vi "launch_main.vi"(8 "error in (no error)":errorcluster, 9 "enable_event":bool, 10 "queue_size":i32=10, 11 "run_f_stop_t":bool) -> (0 "error out":errorcluster, 3 "references":T1)   [LabVIEW 2015, in "repub-dvr_nre.lvlib"]
uses:
  repub-dvr_nre.lvlib
  public/_controls/references.ctl
  _controls/input.ctl
  _controls/input_command.ctl
  _controls/output.ctl
  _controls/data.ctl
  public/_controls/configuration.ctl
  public/_controls/change.ctl
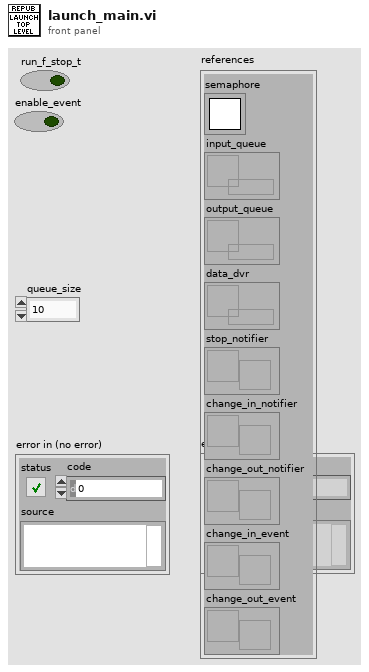
[diagram p1: front panel]
types:
  T1 = typedef "repub-dvr_nre.lvlib/references.ctl" = cluster{"semaphore":T2, "input_queue":refnum<queue>, "output_queue":refnum<queue>, "data_dvr":refnum<data-value>, "stop_notifier":refnum<notifier>, "change_in_notifier":refnum<notifier>, "change_out_notifier":refnum<notifier>, "change_in_event":refnum<user-event>, "change_out_event":refnum<user-event>}
  T2 = typedef "Semaphore RefNum" = refnum<k1>
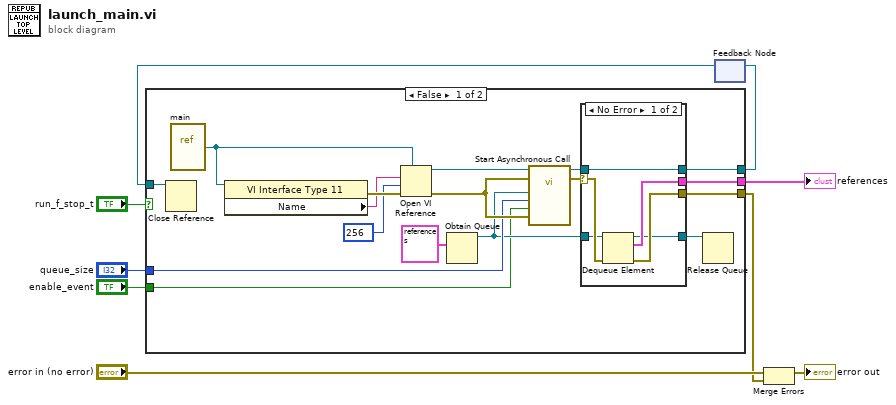
[diagram p0: block diagram]
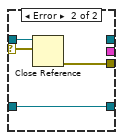
[diagram p2: hidden frame]
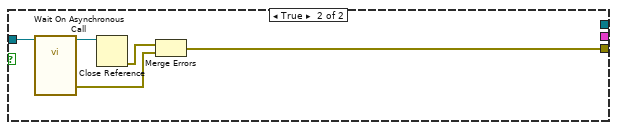
[diagram p3: hidden frame]
diagram:
  n1 = feedback #1() -> (w7:refnum<vi>)  [unwired: 1 in]
  n2 = case shown="False" "run_f_stop_t" {
    tunnel: [w21 _] -> w8
    tunnel: w7 -> [w19 w40]
    tunnel: [w20 w37] -> w5
    tunnel: [w15 _] -> w3
    tunnel: "queue_size" -> [w13 _]
    tunnel: "enable_event" -> [w10 _]
    frame False {
      n3 = Close Reference(reference=w19) -> ()  [unwired: 1 in, 1 out]
      n4 = vi-ref "main.vi"() -> (w18:refnum<vi>)
      n5 = property class="VI Interface Type 11"(reference=w18) -> (error out=w26:errorcluster, "Name"=w25:string)  [unwired: 1 in, 1 out]
      n6 = Open VI Reference(type specifier VI Refnum (for type only)=w18, vi path=w25, options=256, error in (no error)=w26) -> (vi reference=w17:refnum<vi>, error out=w14:errorcluster)  [unwired: 2 in]
      n7 = Obtain Queue(element data type=T1 {"semaphore"=refnum, "input_queue"=refnum, "output_queue"=refnum, "data_dvr"=refnum, "stop_notifier"=refnum, "change_in_notifier"=refnum, "change_out_notifier"=refnum, "change_in_event"=refnum, "change_out_event"=refnum} ("references")) -> (queue out=w12:refnum<queue>)  [unwired: 4 in, 2 out]
      n8 = call-by-ref "Start Asynchronous Call"(reference=w17, error in=w14, 8:"error in (no error)"=w14, "enable_event"=w10, "max_queue_size"=w13, "references_queue"=w12) -> (reference out=w22:refnum<vi>, error out=w23:errorcluster)  [unwired: 7 in, 1 out]
      n9 = case shown="No Error" w23 {
        selector: w23 -> [w32 w35]
        tunnel: [w31 w35] -> w20
        tunnel: w22 -> [w30 w34]
        tunnel: [w30 _] -> w21
        tunnel: w12 -> [w29 w33]
        tunnel: [w28 _] -> w15
        tunnel: [w27 w33] -> w11
        frame No Error {
          n10 = Dequeue Element(queue=w29, error in (no error)=w32) -> (queue out=w27:refnum<queue>, element=w28:T1, error out=w31:errorcluster)  [unwired: 1 in, 1 out]
        }
        frame Error {
          n11 = Close Reference(reference=w34) -> ()  [unwired: 1 in, 1 out]
        }
      }
      n12 = Release Queue(queue=w11) -> ()  [unwired: 2 in, 3 out]
    }
    frame True {
      n13 = call-by-ref "Wait On Asynchronous Call"(reference=w40) -> (reference out=w39:refnum<vi>, "error out"=w36:errorcluster)  [unwired: 12 in, 1 out]
      n14 = Close Reference(reference=w39) -> (error out=w38:errorcluster)  [unwired: 1 in]
      n15 = Merge Errors(w38, w36) -> (w37:errorcluster)
    }
  }
  "references" <- w3
  n16 = feedback-in #1(w8) -> ()
  n17 = Merge Errors("error in (no error)", w5) -> (→"error out":errorcluster)
